vi "Sysdef.SimpleExport.vi"(8 "error in (no error)":errorcluster, 11 "ID":u64) -> (0 "error out":errorcluster, 2 "Export":T1 {"Tree"."Properties"."Type" items=["K_STRING", "K_BOOL", "K_I32", "K_U32", "K_DOUBLE", "K_U64", "K_VARIANT", "K_DEPENDENTFILE", "K_DEPENDENTNODE", "K_DATASOURCENODE", "K_U16", "K_DBLARR", "K_U32ARR", "K_I32ARR", "K_STRINGARR", "K_DICTIONARY", "K_DICTIONARYARR"]}, 3 "ID out":u64)   [LabVIEW 2015, in "System Definition Utilities.lvlib"]
uses:
  System Definition Utilities.lvlib
  _Types/SysDef.Export.ctl
  _Types/TreeItem.ctl
  _Types/TreeItem.Info.ctl
  <vilib>/NI Veristand/Custom Device API/Custom Device Channel.ctl
  <vilib>/NI Veristand/Custom Device API/Custom Device Channel Type.ctl
  <vilib>/NI Veristand/Custom Device API/Custom Device Waveform.ctl
  <vilib>/NI Veristand/Custom Device API/Custom Device Waveform DataType.ctl
  _Types/TreeItem.Property.ctl
  NationalInstruments.VeriStand.SystemDefinitionAPI
  <vilib>/NI VeriStand/Custom Device API/Custom Device API.lvlib
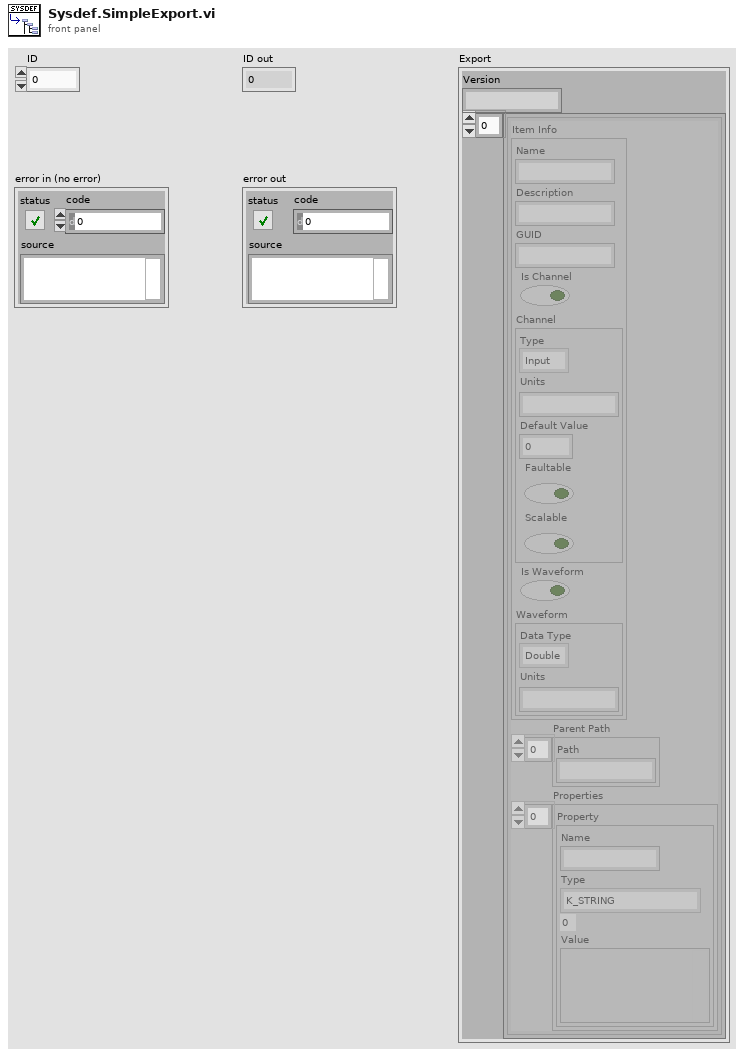
[diagram p1: front panel]
types:
  T1 = typedef "System Definition Utilities.lvlib/SysDef.Export.ctl" = cluster{"Version":string, "Tree":T2[]}
  T2 = typedef "System Definition Utilities.lvlib/TreeItem.ctl" = cluster{"Item Info":T3, "Parent Path":string[], "Properties":T8[]}
  T3 = typedef "System Definition Utilities.lvlib/TreeItem.Info.ctl" = cluster{"Name":string, "Description":string, "GUID":string, "Is Channel":bool, "Channel":T4, "Is Waveform":bool, "Waveform":T6}
  T4 = typedef "Custom Device API.lvlib/Custom Device Channel.ctl" = cluster{"Type":T5, "Units":string, "Default Value":dbl, "Faultable":bool, "Scalable":bool}
  T5 = typedef "Custom Device API.lvlib/Custom Device Channel Type.ctl" = enum16{"Input", "Output"}
  T6 = typedef "Custom Device API.lvlib/Custom Device Waveform.ctl" = cluster{"Data Type":T7, "Units":string}
  T7 = typedef "Custom Device API.lvlib/Custom Device Waveform DataType.ctl" = enum16{"Double", "Complex Double"}
  T8 = typedef "System Definition Utilities.lvlib/TreeItem.Property.ctl" = cluster{"Name":string, "Type":i32, "Value":variant}
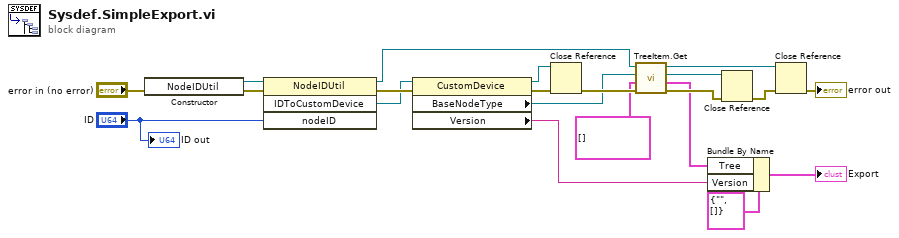
[diagram p0: block diagram]
diagram:
  n1 = constructor class="NodeIDUtil"(error in="error in (no error)") -> (reference out=w16:refnum<k24>, error out=w18:errorcluster)  [unwired: 2 in, 1 out]
  n2 = invoke class="NodeIDUtil" method="IDToCustomDevice"(reference=w16, error in=w18, "nodeID"="ID") -> (reference out=w11:refnum<k24>, error out=w21:errorcluster, "IDToCustomDevice"=w20:refnum<k24>)  [unwired: 1 in, 1 out]
  n3 = property class="CustomDevice"(reference=w20, error in=w21) -> (reference out=w13:refnum<k24>, error out=w15:errorcluster, "BaseNodeType"=w12:refnum<k24>, "Version"=w3:string)
  n4 = Close Reference(reference=w13, error in (no error)=w15) -> (error out=w14:errorcluster)
  n5 = call "TreeItem.Get.vi"("error in (no error)"=w14, "Tree"=T2[] [], "CustomDevice BaseNode Ref"=w12, "NodeIDUtil Ref"=w11) -> ("error out"=w9:errorcluster, "Tree"=w1:T2[], "CustomDevice BaseNode Ref out"=w10:refnum<k24>, "NodeIDUtil Ref out"=w6:refnum<k24>)  [unwired: 4 in]
  n6 = Bundle By Name(cluster=T1 {"Version"="", "Tree"=[]}, "Tree"=w1, "Version"=w3) -> (→"Export":T1)
  n7 = Close Reference(reference=w10, error in (no error)=w9) -> (error out=w8:errorcluster)
  n8 = Close Reference(reference=w6, error in (no error)=w8) -> (error out=→"error out":errorcluster)
  "ID out" <- "ID"
